vi "create command listener schedule.vi"(8 "Comms data in":T1, 11 "RT Queues":T3={"RT Message"=refnum, "RT Comms"=refnum, "RT Data"=refnum, "RT FIFO"=refnum, "message scheduler"=refnum}) -> (0 "Comms data out":T1)   [LabVIEW 2018]
uses:
  <resource>/objmgr/ni.dex.rc
  Chris VIs/Message Scheduler/message scheduler.lvclass
  Type Defs/Queues cluster.ctl
  Type Defs/generic incident.ctl
  comms data.ctl
panel:
  out "schedule ID":u32
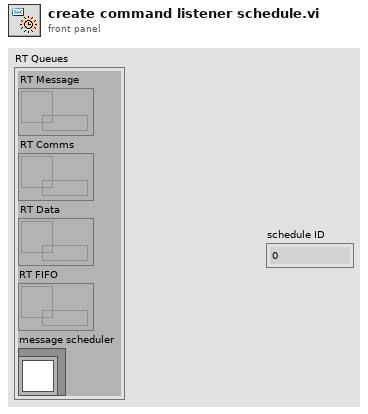
[diagram p1: front panel]
types:
  T1 = typedef "comms data.ctl" = cluster{"Parameters":cluster{"error writer name":string, "command reader name":string, "error buffer size":i32, "command buffer size":i32, "scanivalveIP":string, "scanivalvePeriod":u16}, "Variables":cluster{"listen schedule":u32, "incident buffer":T2[], "command stream":refnum<k21>, "error stream":refnum<k21>, "waiting for command stream connect":bool, "waiting for error stream connect":bool, "scanivalve connection":refnum<k5>, "scanivalveScheduleID":u32}}
  T2 = typedef "generic incident.ctl" = cluster{"timestamp":timestamp, "type":string, "Variant":variant}
  T3 = typedef "Queues cluster.ctl" = cluster{"RT Message":refnum<queue>, "RT Comms":refnum<queue>, "RT Data":refnum<queue>, "RT FIFO":refnum<queue>, "message scheduler":refnum<class "message scheduler.lvclass">}
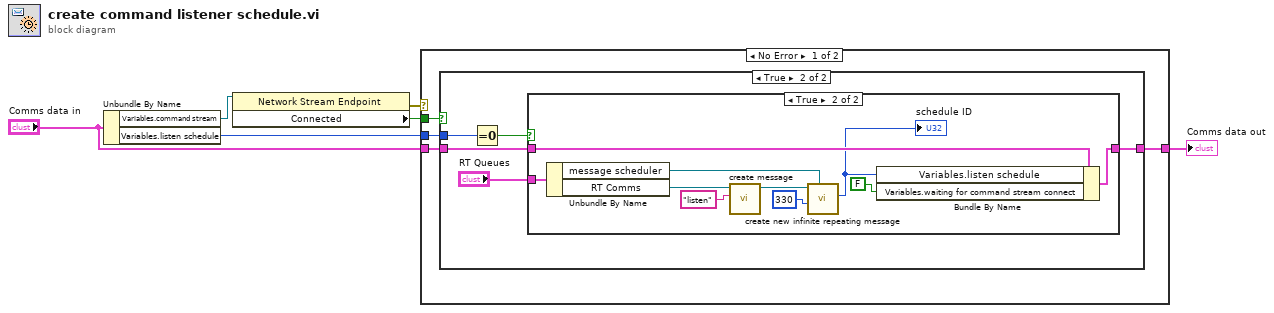
[diagram p0: block diagram]
diagram:
  n1 = Unbundle By Name("Comms data in") -> ("Variables.command stream"=w3:refnum<k21>, "Variables.listen schedule"=w4:u32)
  n2 = property class="Network Stream Endpoint"(reference=w3) -> (error out=w2:errorcluster, "Connected"=w1:bool)  [unwired: 1 in, 1 out]
  n3 = case shown="No Error" w2 {
    tunnel: [w10 w28] -> w6
    tunnel: "Comms data in" -> [w9 w28]
    tunnel: w4 -> [w8 _]
    tunnel: w1 -> [w7 _]
    frame No Error {
      n4 = case shown="True" w7 {
        tunnel: [w11 w15] -> w10
        tunnel: w9 -> [w11 w14]
        tunnel: w8 -> [_ w12]
        frame False {
        }
        frame True {
          n5 = Equal To 0?(x=w12) -> (x = 0?=w13:bool)
          n6 = case shown="True" w13 {
            tunnel: "RT Queues" -> [_ w22]
            tunnel: w14 -> [w17 w21]
            tunnel: [w17 w19] -> w15
            frame False {
            }
            frame True {
              n7 = Unbundle By Name(w22) -> ("message scheduler"=w23:refnum<class "message scheduler.lvclass">, "RT Comms"=w27:refnum<queue>)
              n8 = call "create message.vi"("message"="listen", "queue ref"=w27) -> ("standard message out"=w25:refnum<class "standard message.lvclass">)  [unwired: 8 in, 1 out]
              n9 = call "create new infinite repeating message.vi"("message scheduler"=w23, "ms delay"=u32 330, "message"=w25) -> ("schedule ID"=w18:u32)  [unwired: 7 in, 1 out]
              "schedule ID" <- w18
              n10 = Bundle By Name(cluster=w21, "Variables.listen schedule"=w18, "Variables.waiting for command stream connect"=FALSE) -> (w19:T1)
            }
          }
        }
      }
    }
    frame Error {
    }
  }
  "Comms data out" <- w6
